vi "run action.vi"(7 "first call?":bool, 8 "error in (no error)":errorcluster, 9 "result allocation":T2, 10 "parameters":T2, 11 "action with configuration":T1) -> (0 "error out":errorcluster, 1 "results":T2, 2 "parameters allocation":T2, 3 "action with configuration out":T1, 4 "complete?":bool)   [LabVIEW 2015, in "Simple Sequencer TBM runtime.lvclass"]
doc: "This VI provides each Action with the subset of channel data from the main sequencer that it requested. It then calls the next action, and integrates the action results back into the channel data."
uses:
  Simple Sequencer TBM runtime.lvclass
  <vilib>/NI/Tag Bus/table/data table.ctl
  actions with configuration.ctl
  sequencer parent classes/action parent/action.lvclass
  <vilib>/NI/Tag Bus/table/transfer specification.ctl
  <vilib>/NI/Tag Bus/tag/Data Type.ctl
  <vilib>/NI/Tag Bus/table/data table.lvlib
  <vilib>/NI/Tag Bus/tag/tag descriptor.lvclass
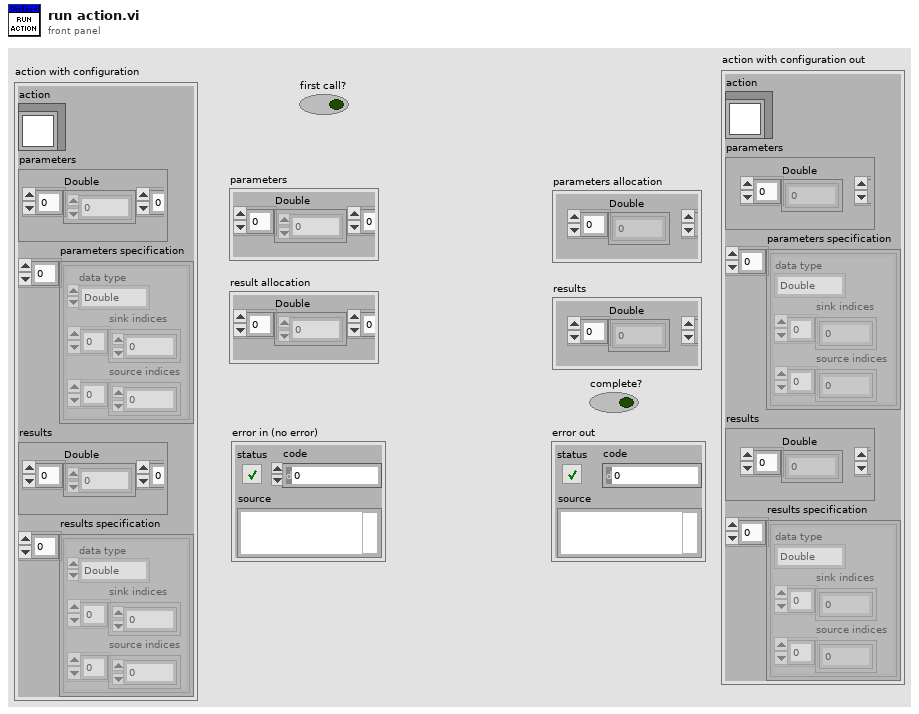
[diagram p1: front panel]
types:
  T1 = typedef "Simple Sequencer TBM runtime.lvclass/actions with configuration.ctl" = cluster{"action":refnum<class "action.lvclass">, "parameters":T2, "parameters specification":T3[], "results":T2, "results specification":T3[]}
  T2 = typedef "tag bus.lvlib/data table.lvlib/data table.ctl" = cluster{"Double":dbl[], "Single":sgl[], "I64":i64[], "I32":i32[], "I16":i16[], "I8":i8[], "U64":u64[], "U32":u32[], "U16":u16[], "U8":u8[], "Boolean":bool[], "String":string[], "Array of Double":cluster{"DBL Array":dbl[]}[], "Array of Single":cluster{"SGL Array":sgl[]}[], "Array of I64":cluster{"I64 Array":i64[]}[], "Array of I32":cluster{"I32 Array":i32[]}[], "Array of I16":cluster{"I16 Array":i16[]}[], "Array of I8":cluster{"I8 Array":i8[]}[], "Array of U64":cluster{"U64 Array":u64[]}[], "Array of U32":cluster{"U32 Array":u32[]}[], "Array of U16":cluster{"U16 Array":u16[]}[], "Array of U8":cluster{"U8 Array":u8[]}[], "Array of Boolean":cluster{"Boolean Array":bool[]}[], "Array of String":cluster{"String Array":string[]}[]}
  T3 = typedef "tag bus.lvlib/data table.lvlib/transfer specification.ctl" = cluster{"data type":T4, "sink indices":i32[], "source indices":i32[]}
  T4 = typedef "tag bus.lvlib/tag descriptor.lvclass/Data Type.ctl" = enum16{"Double", "Single", "I64", "I32", "I16", "I8", "U64", "U32", "U16", "U8", "Boolean", "String", "Array of Double", "Array of Single", "Array of I64", "Array of I32", "Array of I16", "Array of I8", "Array of U64", "Array of U32", "Array of U16", "Array of U8", "Array of Boolean", "Array of String"}
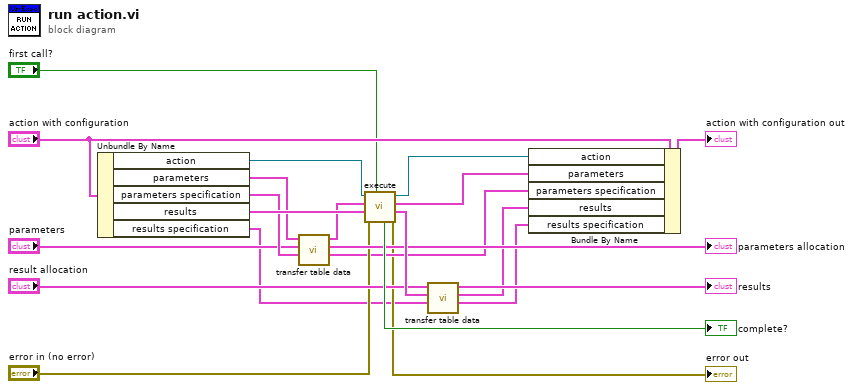
[diagram p0: block diagram]
diagram:
  n1 = Unbundle By Name("action with configuration") -> ("action"=w17:refnum<class "action.lvclass">, "parameters"=w12:T2, "parameters specification"=w16:T3[], "results"=w20:T2, "results specification"=w5:T3[])
  n2 = call <vilib>:"transfer table data.vi"("transfer specification in"=w16, "data table source in"="parameters", "data table sink in"=w12) -> ("transfer specification out"=w7:T3[], "data table source out"=→"parameters allocation":T2, "data table sink out"=w11:T2)  [unwired: 6 in]
  n3 = call-dynamic "execute.vi"("first call?"="first call?", "error in (no error)"="error in (no error)", "result allocation"=w20, "parameters"=w11, "action in"=w17) -> ("error out"=→"error out":errorcluster, "results"=w21:T2, "parameter allocation"=w22:T2, "action out"=w18:refnum<class "action.lvclass">, "complete?"=→"complete?":bool)  [unwired: 2 in]
  n4 = call <vilib>:"transfer table data.vi"("transfer specification in"=w5, "data table source in"=w21, "data table sink in"="result allocation") -> ("transfer specification out"=w4:T3[], "data table source out"=w8:T2, "data table sink out"=→"results":T2)  [unwired: 6 in]
  n5 = Bundle By Name(cluster="action with configuration", "action"=w18, "parameters"=w22, "parameters specification"=w7, "results"=w8, "results specification"=w4) -> (→"action with configuration out":T1)
